vi "Estimate Position.vi"(0 "Intersections":T1(array[cluster])) -> (1 "X":dbl, 2 "Y":dbl)   [LabVIEW 2014, in "Position.lvclass"]
uses:
  Position.lvclass
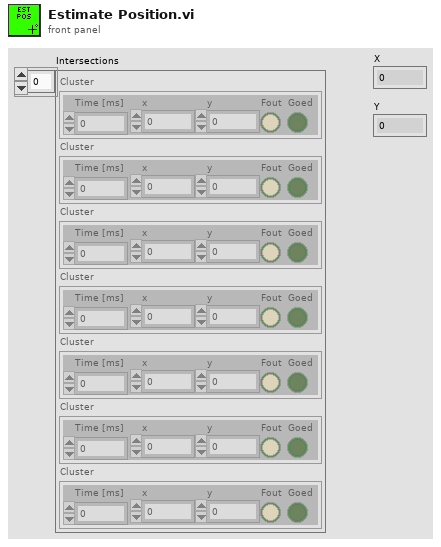
[diagram p1: front panel]
types:
  T1 = cluster{"Time [ms]":dbl, "x":dbl, "y":dbl, "Fout":bool, "Goed":bool}[]
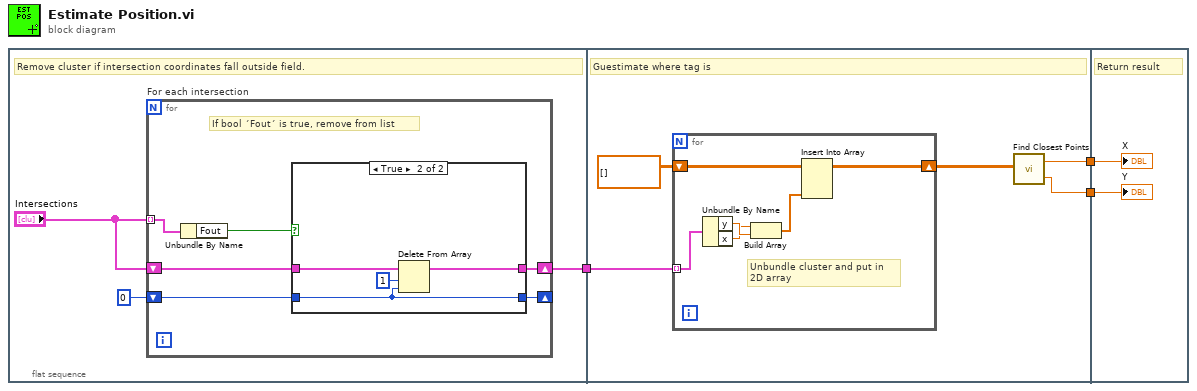
[diagram p0: block diagram]
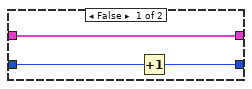
[diagram p2: hidden frame]
diagram:
  n1 = flat-sequence {
    tunnel: [w4] -> w3
    tunnel: w3 -> [w24]
    tunnel: [w21] -> w2
    tunnel: [w20] -> w1
    tunnel: w2 -> [w32]
    tunnel: w1 -> [w31]
    frame #0 {
      # "Remove cluster if intersection coordinates fall outside field."
      n2 = for "For each intersection" {
        tunnel: "Intersections" -> [w9] mode=indexing
        shift-right: [w10] -> w4
        shift-left: "Intersections" -> [w11]
        shift-right: [w7] -> _
        shift-left: 0 -> [w8]
        # "If bool ´Fout´ is true, remove from list"
        n3 = Unbundle By Name "Unbundle By Name"(w9) -> ("Fout"=w12:bool)
        n4 = case shown="True" w12 {
          tunnel: w11 -> [w15 w19]
          tunnel: [w15 w18] -> w10
          tunnel: w8 -> [w14 w16]
          tunnel: [w13 w16] -> w7
          frame False {
            n5 = Increment(x=w14) -> (x+1=w13:i32)
          }
          frame True {
            n6 = Delete From Array(array=w19, length=1, index=w16) -> (array with subset deleted=w18:T1)  [unwired: 1 out]
          }
        }
      }
    }
    frame #1 {
      # "Guestimate where tag is"
      n7 = for {
        tunnel: w24 -> [w30] mode=indexing
        shift-right: [w25] -> w22
        shift-left: dbl[][] [] -> [w29]
        # "Unbundle cluster and put in\n2D array"
        n8 = Unbundle By Name(w30) -> ("y"=w28:dbl, "x"=w27:dbl)
        n9 = Build Array(w27, w28) -> (w26:dbl[])
        n10 = Insert Into Array "Insert Into Array"(array=w29, new element=w26) -> (w25:dbl[][])  [unwired: 2 in]
      }
      n11 = call "Find Closest Points.vi"("Intersection coordinates"=w22) -> ("CenterOfGravityX"=w21:dbl, "CenterOfGravityY"=w20:dbl)
    }
    frame #2 {
      # "Return result"
      "X" <- w32
      "Y" <- w31
    }
  }
